vi "RT Driver VI.vi"(7 "Operation":T1, 11 "Device Reference in":T2 format="%.0x") -> (0 "Error Code":i32)   [LabVIEW 2019, in "FPGA Addon Engine.lvlib"]
uses:
  FPGA Addon Engine.lvlib
  <vilib>/NI VeriStand/Custom Device API/Custom Device Item Ref.ctl
  <vilib>/NI VeriStand/Custom Device API/Hardware Interface Driver VI Operation.ctl
  <vilib>/NI/NIVS Inline Async API/_VS Inline Async API/VS Inline Async API/VS Inline Async API.lvclass/VS Inline Async API.ctl
  <vilib>/NI/NIVS Inline Async API/_Data Access Engine/Data Access Engine/Data Access Engine.lvclass/Data Access Engine.ctl
  <vilib>/NI/NIVS Inline Async API/_Data Access Engine/Access Type Classes/Write/Write.lvclass/Write.ctl
  <vilib>/NI/NIVS Inline Async API/_Data Access Engine/Access Type Classes/ReadWrite/ReadWrite.lvclass/ReadWrite.ctl
  Shared/FPGA Settings.vi
  SubVIs/Initialize Scalar Datatypes and Refs.vi
  <vilib>/NI/NIVS Inline Async API/_Data Access Engine/Data Access Engine/Methods/Data.Engine.Read Data from HW.vi
  <vilib>/NI/NIVS Inline Async API/_VS Inline Async API/Error Handling Process/SubVIs/Error.GetError.vi
  <vilib>/NI/NIVS Inline Async API/_Data Access Engine/Access Type Classes/ReadWrite/ReadWrite.EngineData.vi
  <vilib>/NI/NIVS Inline Async API/_Data Access Engine/Access Type Classes/Write/Write.EngineData.vi
  <vilib>/NI VeriStand/Custom Device API/NI VeriStand - Get Channel Value by Data Reference.vi
  <vilib>/NI VeriStand/Custom Device API/NI VeriStand - Set Channel Value by Data Reference.vi
  <vilib>/Utility/config.llb/Open Config Data.vi
  <vilib>/Utility/config.llb/Get Key Names.vi
  <vilib>/Utility/config.llb/Write Key.vi
  <vilib>/Utility/config.llb/Write Key (I32).vi
  <vilib>/Utility/config.llb/Close Config Data.vi
  Shared/Constants.vi
  <vilib>/NI VeriStand/Custom Device API/NI VeriStand - Get Item Property.vi
  <vilib>/NI VeriStand/Custom Device API/Get Item Property (Variant).vi
  <vilib>/NI VeriStand/Custom Device API/Get Item Property (Dependent File).vi
  <vilib>/NI VeriStand/Custom Device API/Get Item Property (Path).vi
  <vilib>/NI VeriStand/Custom Device API/Get Item Property (String).vi
  <vilib>/NI VeriStand/Custom Device API/NI VeriStand - Set Item Property.vi
  <vilib>/NI VeriStand/Custom Device API/Set Item Property (Path).vi
  <vilib>/NI VeriStand/Custom Device API/Set Item Property (String).vi
  SubVIs/Initialize Input DMA Refs.vi
  SubVIs/Initialize Output DMA Refs.vi
  SubVIs/Initialize Scalar Datatype Classes.vi
  SubVIs/Output DMA Engine.vi
  <vilib>/Utility/error.llb/Error Cluster From Error Code.vi
  <vilib>/RVI Host/nirviSupport.llb/nirviErrorClusterFromErrorCode.vi
  <vilib>/rvi/errors/niLvFpgaAdjustHostInterfaceError.vi
  <vilib>/NI VeriStand/Custom Device API/Global Data Refs.vi
  <vilib>/FPGAPlugInAG/Dynamic/niLvFpga_Close_Dynamic.vi
  <vilib>/NI VeriStand/Custom Device Waveform API/Multiple Waveforms Write (DBL)/Multiple Waveforms Write (DBL).lvclass
  <vilib>/NI VeriStand/Custom Device Waveform API/Single Waveform Read (DBL)/Single Waveform Read (DBL).lvclass
  <vilib>/NI/NIVS Inline Async API/_VS Inline Async API/VS Inline Async API/VS Inline Async API.lvclass
  <vilib>/rvi/interface/nirviMethod/nirviMethod.xnode
  <vilib>/rvi/interface/nirviCloseFPGA/nirviCloseFPGA.xnode
  <vilib>/NI VeriStand/Custom Device API/Custom Device API.lvlib
  <vilib>/NI VeriStand/Custom Device Tools/Custom Device Utility Library/Custom Device Utility Library.lvlib
  <vilib>/rvi/interface/nirviMethod/StockFPGA_InlinedMethodWaitForSingleIRQ.vi
  <vilib>/FPGAPlugInAG/Dynamic/niLvFpga_WaitOnIrq_Dynamic.vi
  <vilib>/FPGAPlugInAG/Dynamic/niLvFpga_AcknowledgeIrq_Dynamic.vi
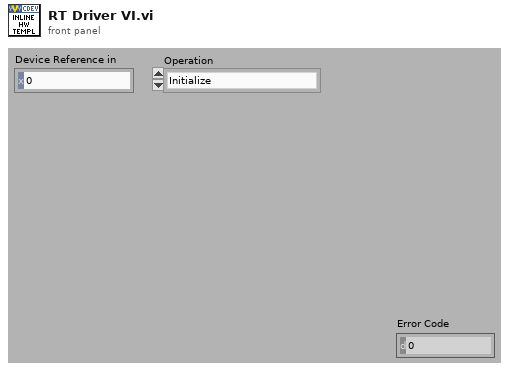
[diagram p1: front panel]
types:
  T1 = typedef "Custom Device API.lvlib/Hardware Interface Driver VI Operation.ctl" = enum16{"Initialize", "Start", "Read Data from HW", "Write Data to HW", "Close"}
  T2 = typedef "Custom Device API.lvlib/Custom Device Item Ref.ctl" = u64
  T3 = typedef "FPGA Addon Engine.lvlib/State Variables.ctl" = cluster{"FPGA Ref":refnum<k20>, "IncomingRegisters.Refs":T4[], "IncomingDMA.Refs":T7[], "OutgoingRegisters.Refs":T4[], "OutgoingDMA.Refs":T12[], "Compiled":T14}
  T4 = typedef "FPGA Addon Engine.lvlib/Register Settings.ctl" = cluster{"Data Type":T5, "U64":refnum<k20>, "U32":refnum<k20>, "U16":refnum<k20>, "U8":refnum<k20>, "I64":refnum<k20>, "I32":refnum<k20>, "I16":refnum<k20>, "I8":refnum<k20>, "SGL":refnum<k20>, "Bool":refnum<k20>, "Scalar Type":T6, "Index":i32, "Length":i32, "Analog PWM In":refnum<k20>, "Digital PWM In":refnum<k20>, "Digital PWM Out":refnum<k20>, "Analog PWM In Settings":refnum<k20>, "Digital PWM In Settings":refnum<k20>, "Sine Out":refnum<k20>, "FXP+/-24.5":refnum<k20>, "FXP+/-16.5":refnum<k20>, "FXP+/-32.8":refnum<k20>, "FXP+/-64.32":refnum<k20>, "FXP+/-16.7":refnum<k20>, "FXP+/-20.5":refnum<k20>, "FXP+/-27.5":refnum<k20>, "FXP+/-32.16":refnum<k20>, "FXP+16.3":refnum<k20>, "FXP+18.3":refnum<k20>, "Digital Static In":refnum<k20>, "Digital Static Out":refnum<k20>, "Digital Static In Settings":refnum<k20>, "Digital WSS Out":refnum<k20>, "Quad Encoder Settings":refnum<k20>, "Quad Encoder In":refnum<k20>}
  T5 = typedef "FPGA Addon Shared.lvlib/Data Type.ctl" = enum8{"<Null>", "I8", "I16", "I32", "I64", "U8", "U16", "U32", "U64", "SGL", "Boolean", "Analog PWM In Settings", "Analog PWM In", "Digital PWM In Settings", "Digital PWM In", "Digital PWM Out", "Sine Out", "FXP+/-24.5", "FXP+/-16.5", "FXP+/-32.8", "FXP+/-64.32", "FXP+/-16.7", "FXP+/-20.5", "FXP+/-27.5", "FXP+/-32.16", "FXP +16.3", "FXP +18.3", "Digital Static In", "Digital Static Out", "Digital Static In Settings", "Digital WSS Out", "Quad Encoder Settings", "Quad Encoder In"}
  T6 = typedef "FPGA Addon Shared.lvlib/Scalar Type.ctl" = enum16{"Standard", "Bitpacked"}
  T7 = typedef "FPGA Addon Engine.lvlib/DMA Input References.ctl" = cluster{"Waveform Ref":refnum<class "Multiple Waveforms Write (DBL).lvclass">, "Name":string, "DMA Settings":T8, "Refs":T11}
  T8 = typedef "FPGA Addon Shared.lvlib/DMA Settings.ctl" = cluster{"Number of Channels":u8, "Delacing Scheme":T9, "Update Rate":u32, "dt":dbl, "Mode":T10, "Number of Samples":u32, "DMA Host Buffer":u32}
  T9 = typedef "FPGA Addon Shared.lvlib/Delacing Scheme.ctl" = enum8{"Interleaved", "Bitpacked"}
  T10 = typedef "FPGA Addon Shared.lvlib/DMA Acquisition Mode.ctl" = enum8{"Continuous", "Triggered Finite"}
  T11 = typedef "FPGA Addon Engine.lvlib/DMA Input Refs.ctl" = cluster{"Data Type":T5, "DMA_SGL":refnum<k20>, "DMA_U64":refnum<k20>, "DMA_I64":refnum<k20>, "DMA_FXP+/-32.8":refnum<k20>, "DMA_FXP+/-64.32":refnum<k20>, "DMA_U32":refnum<k20>, "DMA_U16":refnum<k20>, "DMA_U8":refnum<k20>, "DMA_I32":refnum<k20>, "DMA_I16":refnum<k20>, "DMA_I8":refnum<k20>, "DMA_FXP+/-32.16":refnum<k20>}
  T12 = typedef "FPGA Addon Engine.lvlib/DMA Output References.ctl" = cluster{"Waveforms":refnum<class "Single Waveform Read (DBL).lvclass">[], "Name":string, "Refs":T13}
  T13 = typedef "FPGA Addon Engine.lvlib/DMA Output Refs.ctl" = cluster{"Data Type":T5, "DMA_SGL":refnum<k20>, "DMA_U64":refnum<k20>, "DMA_I64":refnum<k20>, "DMA_FXP+/-32.8":refnum<k20>, "DMA_FXP+/-64.32":refnum<k20>, "DMA_U32":refnum<k20>, "DMA_U16":refnum<k20>, "DMA_U8":refnum<k20>, "DMA_I32":refnum<k20>, "DMA_I16":refnum<k20>, "DMA_I8":refnum<k20>, "DMA_FXP+/-32.16":refnum<k20>}
  T14 = typedef "FPGA Addon Shared.lvlib/Compiled.Settings.ctl" = cluster{"Name":string, "IncomingRegisters.Settings":T15[], "IncomingRegisters.Refs":cluster{"Refs":T17[], "Values":dbl[]}, "OutgoingRegisters.Settings":T15[], "OutgoingRegisters.Refs":cluster{"Refs":T17[], "Values":dbl[]}, "Incoming.Size":i32, "Outgoing.Size":i32, "IncomingDMA.Settings":T19[], "OutgoingDMA.Settings":T19[], "FPGA.Settings":T21, "Target.Type":T22}
  T15 = typedef "FPGA Addon Shared.lvlib/Compiled.RegisterSettings.ctl" = cluster{"Scalar Type":T6, "Index":i32, "Length":i32, "Register":T16}
  T16 = typedef "FPGA Addon Shared.lvlib/Register Information.ctl" = cluster{"Name":string, "Data Type":T5, "Default Value":variant}
  T17 = typedef "Custom Device API.lvlib/Block Data Reference.ctl" = cluster{"Data Reference":T18, "Offset":u64, "Length":u64}
  T18 = typedef "Custom Device API.lvlib/Data Reference.ctl" = i32
  T19 = typedef "FPGA Addon Shared.lvlib/Compiled.DMASettings.ctl" = cluster{"Name":string, "Data Type":T5, "DMA.Settings":T8, "DMA.VSRefs":T20[]}
  T20 = typedef "Custom Device API.lvlib/Waveform Data Reference.ctl" = i32
  T21 = typedef "FPGA Addon Shared.lvlib/FPGA Settings.ctl" = cluster{"Bitfile path":path, "RIO Device Address":string}
  T22 = typedef "Custom Device API.lvlib/Custom Device Target Type.ctl" = enum16{"PharLap", "VxWorks", "Windows", "Linux_32_ARM", "Linux_x64"}
  T23 = cluster{"Vars":T3, "Async?":bool, "Async":refnum<class "VS Inline Async API.lvclass">, "error out":errorcluster}
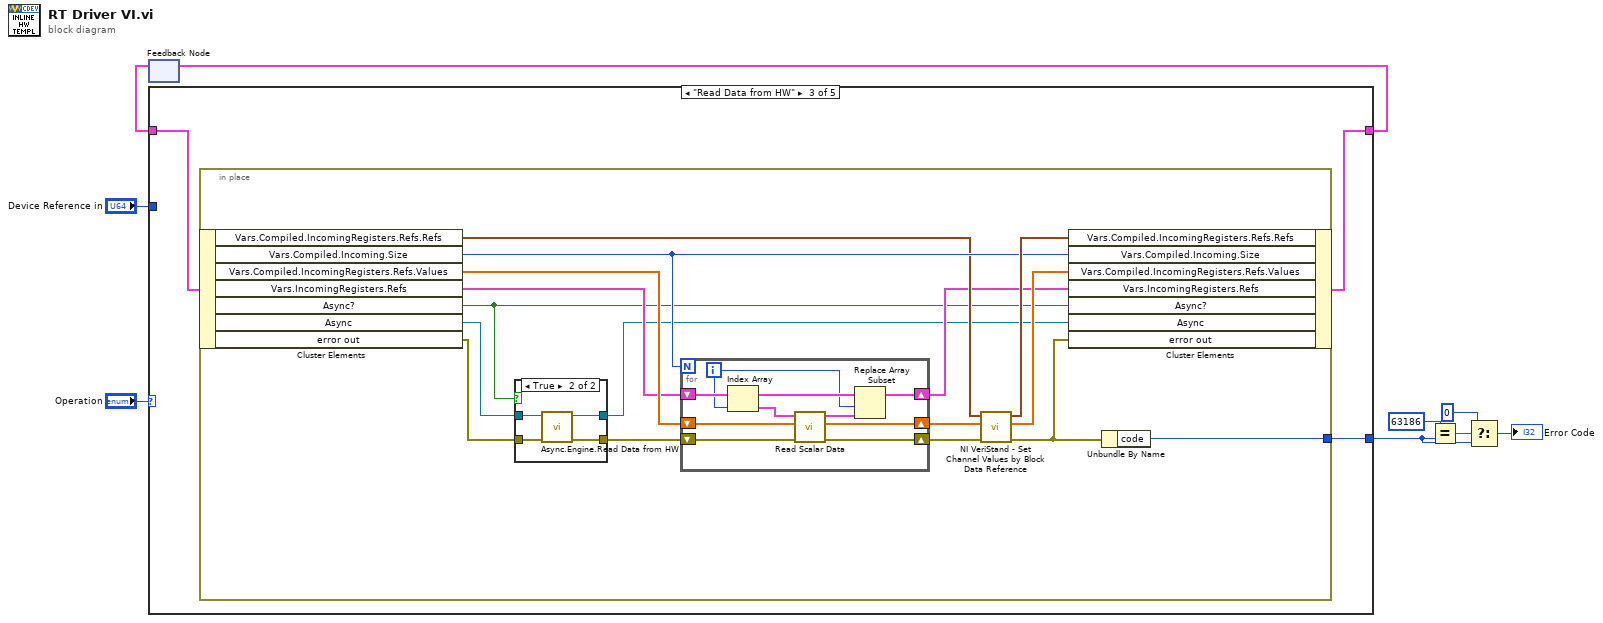
[diagram p0: block diagram]
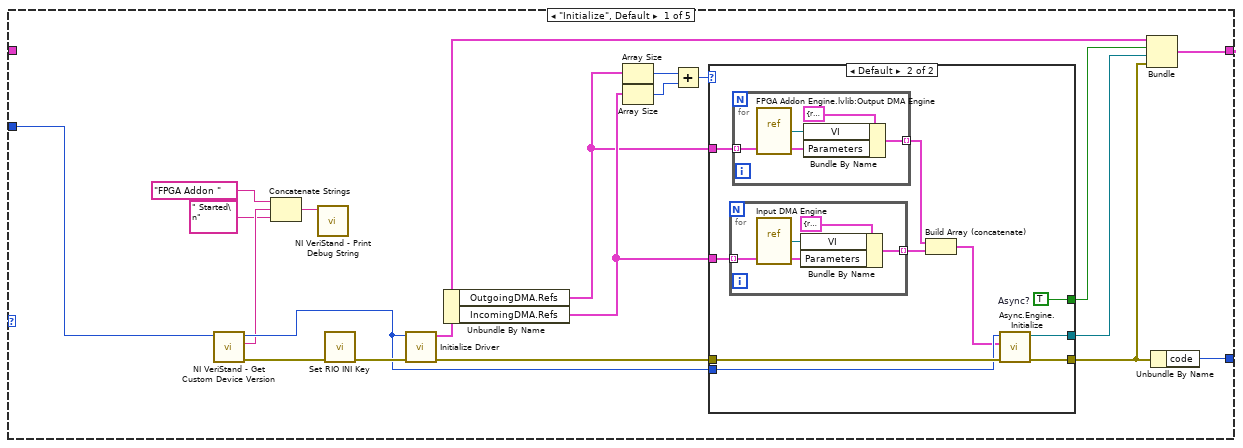
[diagram p2: hidden frame]
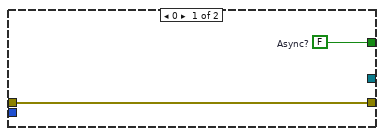
[diagram p3: hidden frame]
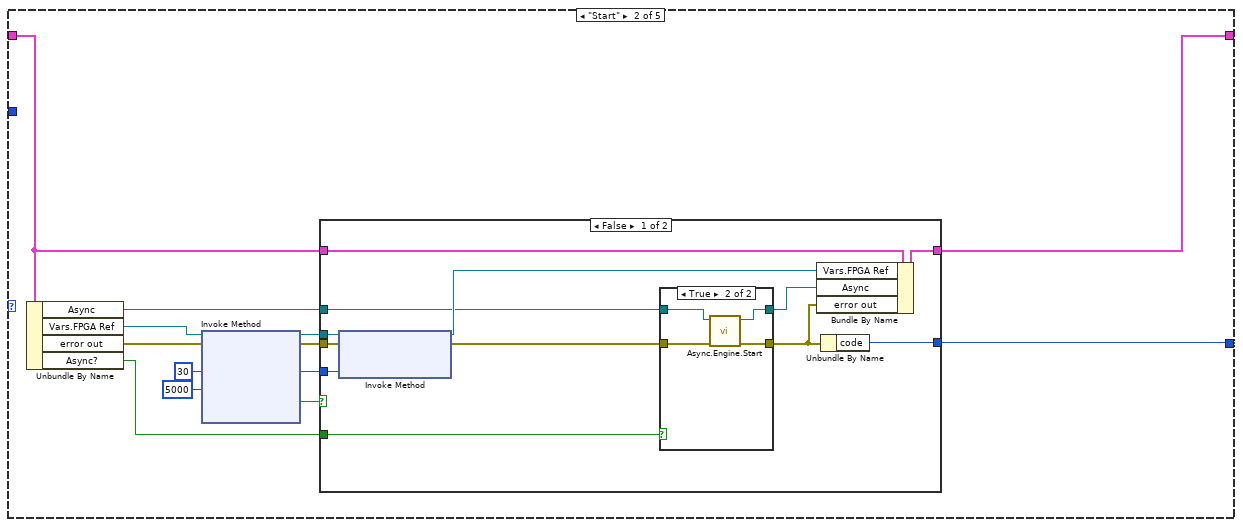
[diagram p4: hidden frame]
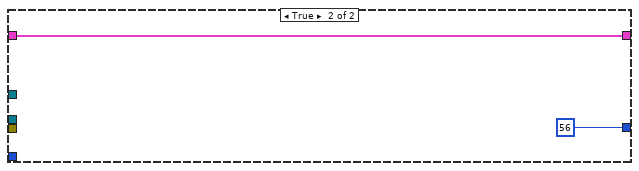
[diagram p6: hidden frame]
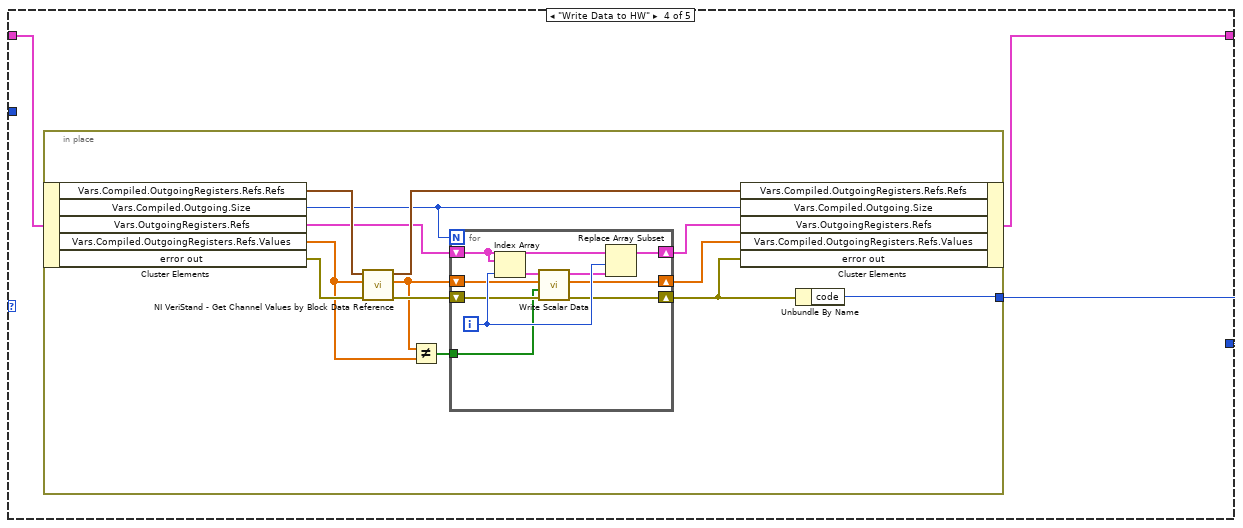
[diagram p8: hidden frame]
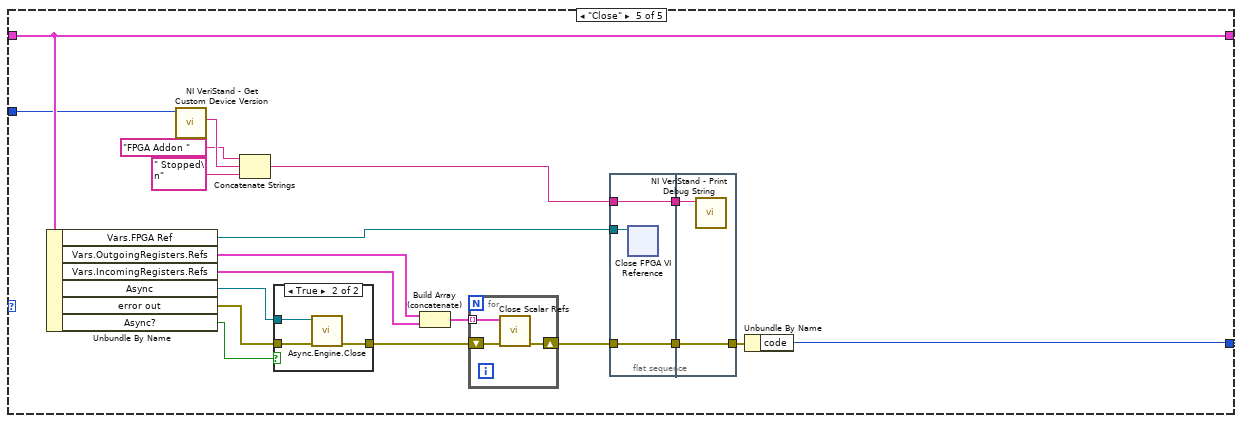
[diagram p9: hidden frame]
diagram:
  n1 = feedback #1() -> (w7:T23)  [unwired: 1 out]
  n2 = case shown="\"Read Data from HW\"" "Operation" {
    tunnel: [w29 w59 w84 w117 w158] -> w8
    tunnel: w7 -> [_ w60 w82 w118 w158]
    tunnel: "Device Reference in" -> [w15 _ _ _ w142]
    tunnel: [w28 w61 w83 w116 w160] -> w3
    frame "Initialize", Default {
      n3 = call <vilib>:"NI VeriStand - Get Custom Device Version.vi"("Device Ref in"=w15) -> ("error out"=w16:errorcluster, "Value"=w13:string, "Device Ref out"=w14:T2)  [unwired: 8 in]
      n4 = Concatenate Strings("FPGA Addon ", w13, " Started\n" ("string")) -> (w10:string)
      n5 = call <vilib>:"NI VeriStand - Print Debug String.vi"("Message"=w10) -> ()  [unwired: 10 in, 1 out]
      n6 = call "Set RIO INI Key.vi"("error in (no error)"=w16) -> ("error out"=w27:errorcluster)  [unwired: 10 in]
      n7 = call "Initialize Driver.vi"("error in (no error)"=w27, "Section Ref in"=w14) -> ("error out"=w26:errorcluster, "Vars"=w17:T3)  [unwired: 8 in]
      n8 = Unbundle By Name(w17) -> ("OutgoingDMA.Refs"=w22:T12[], "IncomingDMA.Refs"=w23:T7[])
      n9 = Array Size(array=w22) -> (size(s)=w21:i32)
      n10 = Array Size(array=w23) -> (size(s)=w20:i32)
      n11 = Add(x=w21, y=w20) -> (x+y=w19:i32)
      n12 = case shown="Default" w19 {
        tunnel: w26 -> [w31 w38]
        tunnel: [w31 w37] -> w25
        tunnel: [_ w36] -> w24
        tunnel: w23 -> [_ w34]
        tunnel: w22 -> [_ w41]
        tunnel: [w30 w39] -> w18
        tunnel: w14 -> [_ w35]
        frame 0 {
          w30 = FALSE  # Async?
        }
        frame Default {
          w39 = TRUE  # Async?
          n13 = for {
            tunnel: w34 -> [w44] mode=indexing
            tunnel: [w43] -> w33 mode=indexing
            n14 = vi-ref "Input DMA Engine.vi"() -> (w42:refnum<vi>)
            n15 = Bundle By Name(cluster=cluster{"VI":refnum<vi>, "Parameters":variant} {"VI"=refnum, "Parameters"=variant} ("Process"), "VI"=w42, "Parameters"=w44) -> (w43:cluster{"VI":refnum<vi>, "Parameters":variant})
          }
          n16 = for {
            tunnel: w41 -> [w48] mode=indexing
            tunnel: [w47] -> w40 mode=indexing
            n17 = vi-ref "FPGA Addon Engine.lvlib:Output DMA Engine.vi"() -> (w46:refnum<vi>)
            n18 = Bundle By Name(cluster=cluster{"VI":refnum<vi>, "Parameters":variant} {"VI"=refnum, "Parameters"=variant} ("Process"), "VI"=w46, "Parameters"=w48) -> (w47:cluster{"VI":refnum<vi>, "Parameters":variant})
          }
          n19 = Build Array (concatenate)(w40, w33) -> (w32:cluster{"VI":refnum<vi>, "Parameters":variant}[])
          n20 = call <vilib>:"Async.Engine.Initialize.vi"("error in (no error)"=w38, "Processes"=w32, "Custom Device Ref"=w35) -> ("error out"=w37:errorcluster, "Async"=w36:refnum<class "VS Inline Async API.lvclass">)  [unwired: 7 in]
        }
      }
      n21 = Bundle("Vars"=w17, "Async?"=w18, "Async"=w24, "error out"=w25) -> (w29:T23)  [unwired: 1 out]
      n22 = Unbundle By Name(w25) -> ("code"=w28:i32)
    }
    frame "Start" {
      w54 = 30 ("IRQ Number(s)")
      n23 = Unbundle By Name(w60) -> ("Async"=w50:refnum<class "VS Inline Async API.lvclass">, "Vars.FPGA Ref"=w58:refnum<k20>, "error out"=w57:errorcluster, "Async?"=w52:bool)
      n24 = xnode "Invoke Method"("FPGA VI Reference In"=w58, "error in"=w57, "IRQ Number(s)"=w54, "Timeout (ms)"=5000) -> ("FPGA VI Reference Out"=w56:refnum<k20>, "error out"=w55:errorcluster, "Timed Out"=w51:bool)  [unwired: 1 out]
      n25 = case shown="False" w51 {
        tunnel: [w73 56 ("code")] -> w61
        tunnel: w60 -> [w72 w81]
        tunnel: [w71 w81] -> w59
        tunnel: w56 -> [w70 _]
        tunnel: w55 -> [w69 _]
        tunnel: w54 -> [w68 _]
        tunnel: w52 -> [w65 _]
        tunnel: w50 -> [w64 _]
        frame False {
          n26 = xnode "Invoke Method"("FPGA VI Reference In"=w70, "error in"=w69, "IRQ Number(s)"=w68) -> ("FPGA VI Reference Out"=w67:refnum<k20>, "error out"=w62:errorcluster)
          n27 = case shown="True" w65 {
            tunnel: w62 -> [w75 w79]
            tunnel: [w75 w78] -> w66
            tunnel: w64 -> [w74 w77]
            tunnel: [w74 w76] -> w63
            frame False {
            }
            frame True {
              n28 = call <vilib>:"Async.Engine.Start.vi"("error in (no error)"=w79, "VS Inline Async API in"=w77) -> ("error out"=w78:errorcluster, "VS Inline Async API out"=w76:refnum<class "VS Inline Async API.lvclass">)  [unwired: 8 in]
            }
          }
          n29 = Bundle By Name(cluster=w72, "Vars.FPGA Ref"=w67, "Async"=w63, "error out"=w66) -> (w71:T23)
          n30 = Unbundle By Name(w66) -> ("code"=w73:i32)
        }
        frame True {
        }
      }
    }
    frame "Read Data from HW" {
      n31 = in-place {
        in-place-border: [w90] -> w83
        n32 = in-place-cluster #2(w82) -> ("Vars.Compiled.IncomingRegisters.Refs.Refs"=w94:T17[], "Vars.Compiled.Incoming.Size"=w96:i32, "Vars.Compiled.IncomingRegisters.Refs.Values"=w100:dbl[], "Vars.IncomingRegisters.Refs"=w93:T4[], "Async?"=w85:bool, "Async"=w87:refnum<class "VS Inline Async API.lvclass">, "error out"=w89:errorcluster)
        n33 = case shown="True" w85 {
          tunnel: w89 -> [w102 w106]
          tunnel: w87 -> [w101 w105]
          tunnel: [w102 w104] -> w88
          tunnel: [w101 w103] -> w86
          frame False {
          }
          frame True {
            n34 = call <vilib>:"Async.Engine.Read Data from HW.vi"("error in"=w106, "Async in"=w105) -> ("error out"=w104:errorcluster, "Async out"=w103:refnum<class "VS Inline Async API.lvclass">)  [unwired: 8 in]
          }
        }
        n35 = for {
          N: w96 -> [_]
          shift-right: [w107] -> w97
          shift-left: w100 -> [w108]
          shift-right: [w115] -> w92
          shift-left: w93 -> [w114]
          shift-right: [w112] -> w95
          shift-left: w88 -> [w113]
          i -> [w109]
          n36 = Index Array(array=w114, index=w109) -> (element=w110:T4)
          n37 = call "Read Scalar Data.vi"("error in (no error)"=w113, "Values"=w108, "Cluster"=w110) -> ("error out"=w112:errorcluster, "Values"=w107:dbl[], "Cluster"=w111:T4)  [unwired: 6 in]
          n38 = Replace Array Subset(array=w114, new element=w111, index=w109) -> (w115:T4[])
        }
        n39 = call <vilib>:"NI VeriStand - Set Channel Values by Block Data Reference.vi"("error in (no error)"=w95, "Values Array in"=w97, "Block Data Ref"=w94) -> ("error out"=w91:errorcluster, "Values Array out"=w98:dbl[], "Block Data Ref dup"=w99:T17[])  [unwired: 6 in]
        n40 = in-place-cluster #2("Vars.Compiled.IncomingRegisters.Refs.Refs"=w99, "Vars.Compiled.Incoming.Size"=w96, "Vars.Compiled.IncomingRegisters.Refs.Values"=w98, "Vars.IncomingRegisters.Refs"=w92, "Async?"=w85, "Async"=w86, "error out"=w91) -> (w84:T23)
        n41 = Unbundle By Name(w91) -> ("code"=w90:i32)
      }
    }
    frame "Write Data to HW" {
      n42 = in-place {
        in-place-border: [w122] -> w116
        n43 = in-place-cluster #3(w118) -> ("Vars.Compiled.OutgoingRegisters.Refs.Refs"=w131:T17[], "Vars.Compiled.Outgoing.Size"=w125:i32, "Vars.OutgoingRegisters.Refs"=w129:T4[], "Vars.Compiled.OutgoingRegisters.Refs.Values"=w120:dbl[], "error out"=w124:errorcluster)
        n44 = call <vilib>:"NI VeriStand - Get Channel Values by Block Data Reference.vi"("error in (no error)"=w124, "Values Array in"=w120, "Block Data Ref"=w131) -> ("error out"=w126:errorcluster, "Values Array out"=w121:dbl[], "Block Data Ref dup"=w130:T17[])  [unwired: 6 in]
        n45 = Not Equal?(x=w121, y=w120) -> (x != y?=w119:bool[])
        n46 = for {
          N: w125 -> [_]
          shift-right: [w133] -> w127
          shift-left: w121 -> [w134]
          shift-right: [w141] -> w128
          shift-left: w129 -> [w140]
          shift-right: [w136] -> w123
          shift-left: w126 -> [w137]
          tunnel: w119 -> [w132]
          i -> [w139]
          n47 = Index Array(array=w140, index=w139) -> (element=w135:T4)
          n48 = call "Write Scalar Data.vi"("error in (no error)"=w137, "Changed?"=w132, "Values"=w134, "Cluster"=w135) -> ("error out"=w136:errorcluster, "Values"=w133:dbl[], "Cluster"=w138:T4)  [unwired: 5 in]
          n49 = Replace Array Subset(array=w140, new element=w138, index=w139) -> (w141:T4[])
        }
        n50 = in-place-cluster #3("Vars.Compiled.OutgoingRegisters.Refs.Refs"=w130, "Vars.Compiled.Outgoing.Size"=w125, "Vars.OutgoingRegisters.Refs"=w128, "Vars.Compiled.OutgoingRegisters.Refs.Values"=w127, "error out"=w123) -> (w117:T23)
        n51 = Unbundle By Name(w123) -> ("code"=w122:i32)
      }
    }
    frame "Close" {
      n52 = Unbundle By Name(w158) -> ("Vars.FPGA Ref"=w150:refnum<k20>, "Vars.OutgoingRegisters.Refs"=w157:T4[], "Vars.IncomingRegisters.Refs"=w156:T4[], "Async"=w147:refnum<class "VS Inline Async API.lvclass">, "error out"=w155:errorcluster, "Async?"=w149:bool)
      n53 = call <vilib>:"NI VeriStand - Get Custom Device Version.vi"("Device Ref in"=w142) -> ("Value"=w146:string)  [unwired: 8 in, 2 out]
      n54 = Concatenate Strings("FPGA Addon ", w146, " Stopped\n" ("string")) -> (w143:string)
      n55 = case shown="True" w149 {
        tunnel: w155 -> [w161 w164]
        tunnel: [w161 w163] -> w154
        tunnel: w147 -> [_ w162]
        frame False {
        }
        frame True {
          n56 = call <vilib>:"Async.Engine.Close.vi"("error in (no error)"=w164, "Async in"=w162) -> ("error out"=w163:errorcluster)  [unwired: 8 in, 1 out]
        }
      }
      n57 = Build Array (concatenate)(w157, w156) -> (w159:T4[])
      n58 = for {
        tunnel: w159 -> [w170] mode=indexing
        shift-right: [w171] -> w148
        shift-left: w154 -> [w172]
        n59 = call "Close Scalar Refs.vi"("error in (no error)"=w172, "Cluster"=w170) -> ("error out"=w171:errorcluster)  [unwired: 9 in]
      }
      n60 = flat-sequence {
        tunnel: w143 -> [w166]
        tunnel: w148 -> [w167]
        tunnel: [w167] -> w152
        tunnel: [w166] -> w151
        tunnel: w150 -> [w165]
        tunnel: [w169] -> w153
        tunnel: w152 -> [w169]
        tunnel: w151 -> [w168]
        frame #0 {
          n61 = xnode "Close FPGA VI Reference"("FPGA VI Reference In"=w165) -> ()  [unwired: 1 in, 1 out]
        }
        frame #1 {
          n62 = call <vilib>:"NI VeriStand - Print Debug String.vi"("Message"=w168) -> ()  [unwired: 10 in, 1 out]
        }
      }
      n63 = Unbundle By Name(w153) -> ("code"=w160:i32)
    }
  }
  n64 = feedback-in #1(w8) -> ()
  n65 = Equal?(x=63186 ("code"), y=w3) -> (x = y?=w4:bool)
  n66 = Select(t=0, s=w4, f=w3) -> (s? t:f=→"Error Code":i32)
